vi "H5D_write_init_cluster.vi"(5 "overwrite?":bool, 6 "preserve attribs?":bool, 7 "dims":i32[](array[numeric]), 8 "element":T1 {"Estimate Source" items=["Basic Labview Estimate", "IDL Estimate"]}, 9 "name":string, 10 "ref":i32) -> (0 "error out":errorcluster, 1 "space":i32, 2 "dtype":i32, 3 "ds_id":i32, 4 "attribs":variant[](array[variant]))   [LabVIEW 2011]
uses:
  Public API/Query_Dust_Event.ctl
  Estimate_source.ctl
  <vilib>/addons/h5labview/H5_errcode.vi
  <vilib>/Utility/error.llb/Error Cluster From Error Code.vi
  <vilib>/addons/_h5labview_internal_deps/hdf5dll.dll
  <vilib>/addons/h5labview/H5Attrib.lvlib
  <vilib>/addons/h5labview/H5Base.lvlib
  <vilib>/addons/h5labview/H5TypeSpace.lvlib
panel:
  # "Dust Event"
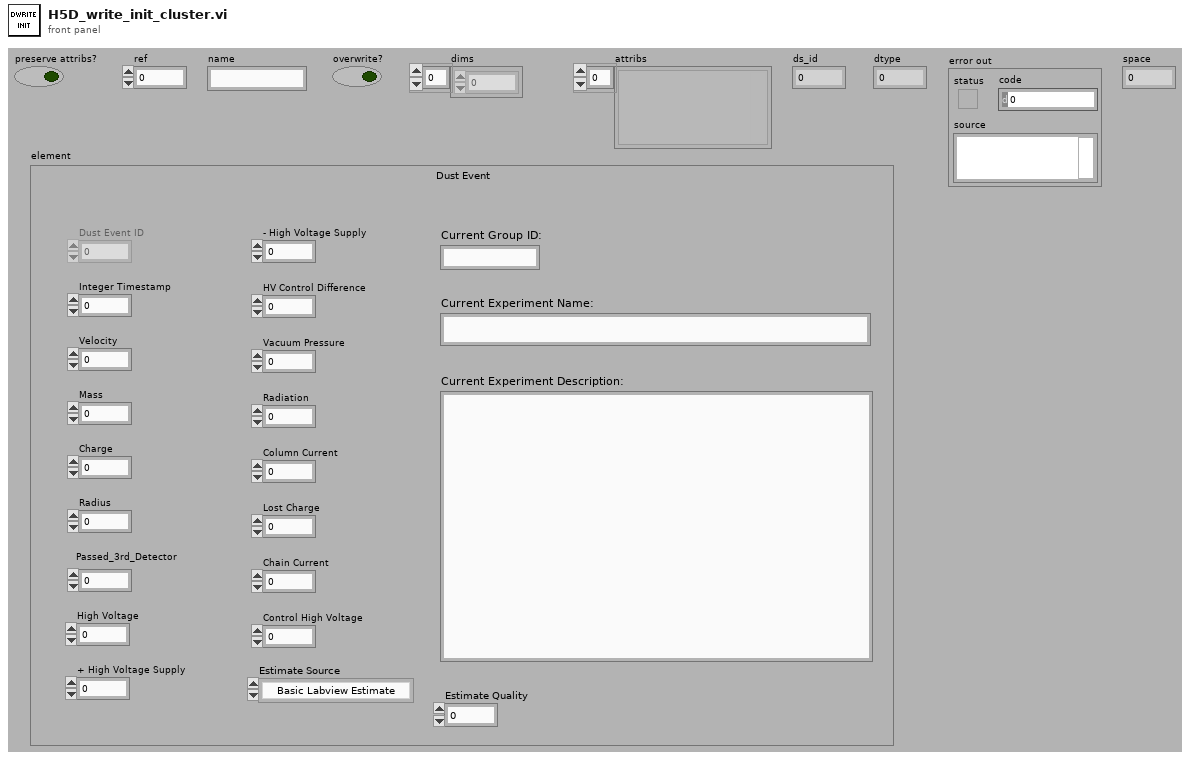
[diagram p1: front panel]
types:
  T1 = typedef "Query_Dust_Event.ctl" = cluster{"Dust Event ID":i64, "Integer Timestamp":i64, "Velocity":sgl, "Mass":sgl, "Charge":sgl, "Radius":sgl, "Passed_3rd_Detector":i8, "High Voltage":sgl, "+ High Voltage Supply":sgl, "- High Voltage Supply":sgl, "HV Control Difference":sgl, "Vacuum Pressure":sgl, "Radiation":sgl, "Column Current":sgl, "Lost Charge":sgl, "Chain Current":sgl, "Control High Voltage":sgl, "Current Group ID:":string, "Current Experiment Name:":string, "Current Experiment Description:":string, "Estimate Source":T2, "Estimate Quality":sgl}
  T2 = typedef "Estimate_source.ctl" = i8
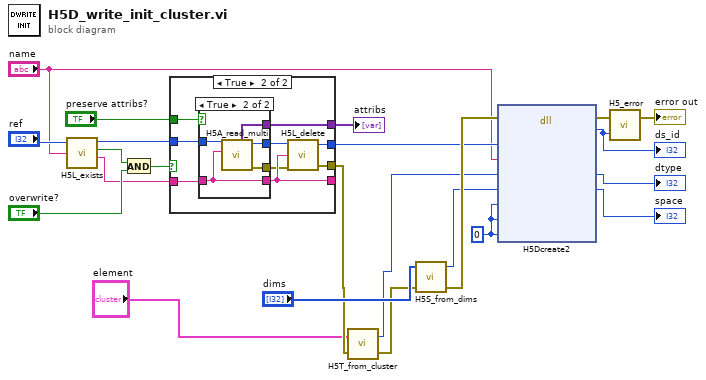
[diagram p0: block diagram]
diagram:
  w9 = 0 ("dapl_id")
  n1 = call <vilib>:"H5L_exists.vi"("path"="name", "loc_id"="ref") -> ("path out"=w13:string, "exists?"=w17:bool, "loc_id out"=w15:i32)  [unwired: 1 in, 1 out]
  n2 = And(x=w17, y="overwrite?") -> (x .and. y?=w14:bool)
  n3 = case shown="True" w14 {
    tunnel: w13 -> [w25 w34]
    tunnel: [w25 w30] -> _
    tunnel: [_ w33] -> w10
    tunnel: "preserve attribs?" -> [_ w32]
    tunnel: w15 -> [w24 w29]
    tunnel: [w24 w28] -> w18
    tunnel: [_ w26] -> w4
    frame False {
    }
    frame True {
      n4 = case shown="True" w32 {
        tunnel: w34 -> [w36 w41]
        tunnel: [w35 w40] -> w31
        tunnel: [_ w39] -> w33
        tunnel: [w36 w41] -> w30
        tunnel: w29 -> [w35 w38]
        tunnel: [_ w37] -> w27
        frame False {
        }
        frame True {
          n5 = call <vilib>:"H5A_read_multi.vi"("obj_name"=w41, "ref"=w38) -> ("error out"=w37:errorcluster, "ref out"=w40:i32, "attribs"=w39:variant[])  [unwired: 5 in]
        }
      }
      n6 = call <vilib>:"H5L_delete.vi"("error in (no error)"=w27, "obj_name"=w30, "loc_id"=w31) -> ("error out"=w26:errorcluster, "loc_id out"=w28:i32)  [unwired: 1 in]
    }
  }
  "attribs" <- w10
  n7 = call <vilib>:"H5T_from_cluster.vi"("error in"=w4, "cluster_in"="element") -> ("error out"=w3:errorcluster, "type_id"=w2:i32)
  n8 = call <vilib>:"H5S_from_dims.vi"("error in (no error)"=w3, "dims"="dims") -> ("error out"=w22:errorcluster, "h5space"=w21:i32)  [unwired: 2 in]
  n9 = dll-call lib="C:/Program Files/National Instruments/LabVIEW 2011/vi.lib/addons/_h5labview_internal_deps/hdf5dll.dll" fn="H5Dcreate2" ("hdf5_call")(error in=w22, "loc_id"=w18, "name"="name", "dtype"=w2, "space"=w21, "lcpl_id"=w9, "dcpl_id"=w9, "dapl_id"=w9) -> (error out=w8:errorcluster, "return type"=w6:i32, "dtype"=→"dtype":i32, "space"=→"space":i32)  [unwired: 7 in, 1 out]
  "ds_id" <- w6
  n10 = call <vilib>:"H5_error.vi"("retval"=w6, "error in (no error)"=w8) -> ("error out"=→"error out":errorcluster)  [unwired: 1 out]
